vi "Convert String to HexString.vi"(1 "String":string) -> (0 "HexString":string)   [LabVIEW 2013]
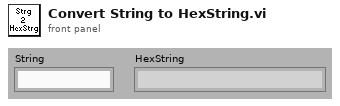
[diagram p1: front panel]
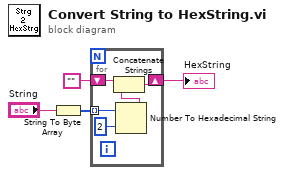
[diagram p0: block diagram]
diagram:
  n1 = String To Byte Array(string="String") -> (unsigned byte array=w1:u8[])
  n2 = for {
    shift-right: [w5] -> w4
    shift-left: "" -> [w7]
    tunnel: w1 -> [w8] mode=indexing
    n3 = Number To Hexadecimal String(1:i16 2 ("width (-)"), 2:w8) -> (0:w6:string)
    n4 = Concatenate Strings(w7, w6) -> (w5:string)
  }
  "HexString" <- w4
